vi "Do.vi"(8 "error in":errorcluster, 10 "Actor in":refnum<class "Actor.lvclass">, 11 "Stop Calibration":refnum<class "Send Stop Calibration MSG.lvclass">) -> (0 "error out":errorcluster, 2 "Actor out":refnum<class "Actor.lvclass">)   [LabVIEW 2014, in "Controller.lvlib" / "Send Stop Calibration MSG.lvclass"]
doc: "(<B>Filename</B>: Actor Framework.lvlib:Message.lvclass:Do.vi)\n\nDefines what a message does when it is received by an actor. Generally, a message instructs an actor to invoke one of its methods. By default, this method does nothing. A child class must override it to define behavior. Create a child class by using the Actor Framework Message Maker dialog box."
uses:
  Send Stop Calibration MSG.lvclass
  <vilib>/ActorFramework/Actor/Actor.lvclass
  Controller.lvclass
  Calibration/Send External Stop MSG/Send External Stop MSG.lvclass
  Controls/eMap.ctl
  <vilib>/ActorFramework/Message Enqueuer/Message Enqueuer.lvclass
  SuperActor/SuperActor.lvclass/SuperActor.ctl
  <vilib>/ActorFramework/Message Enqueuer/Message Enqueuer.lvclass/Message Enqueuer.ctl
  SuperActor/Read Log Session.vi
  <vilib>/ActorFramework/Message Priority Queue/Priority Enqueue.vi
  <userlib>/_Session Fwk/Session - Root.lvclass
  reusable/Session APIs/Session Log/System Log.lvclass
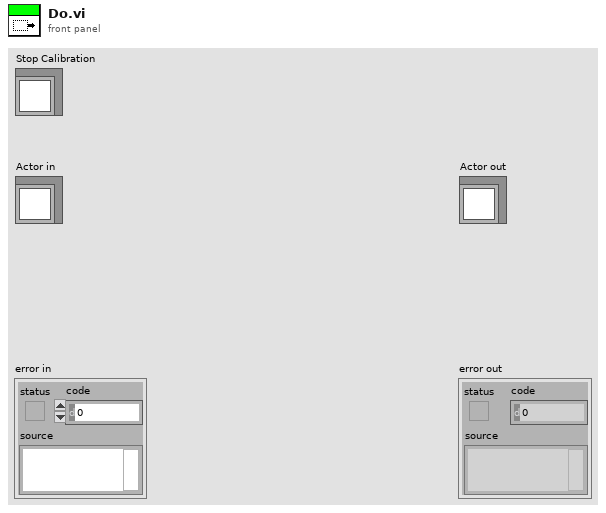
[diagram p1: front panel]
types:
  T1 = typedef "Controller.lvlib/Controller.lvclass/eMap.ctl" = cluster{"Enqueuer":refnum<class "Message Enqueuer.lvclass">, "Active":bool}
  T2 = typedef "Session - Root.lvclass/Session Handle.ctl" = refnum<data-value>
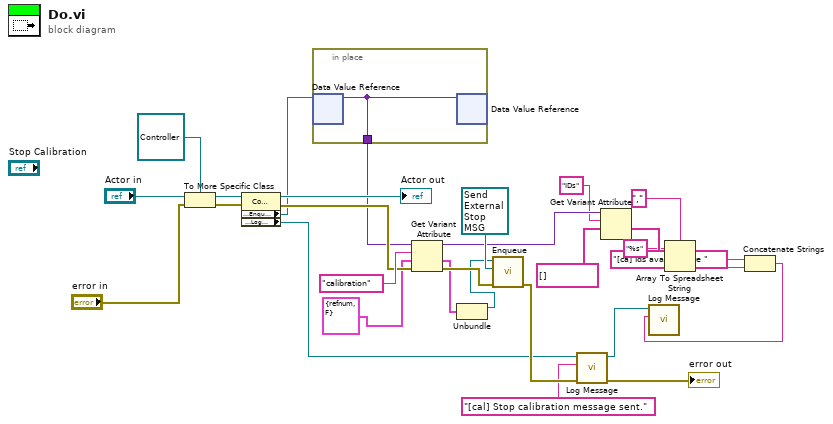
[diagram p0: block diagram]
diagram:
  n1 = To More Specific Class(target class=refnum<class "Controller.lvclass"> refnum ("Controller:Controller"), reference="Actor in", error in="error in") -> (specific class reference=w26:refnum<class "Controller.lvclass">, error out=w24:errorcluster)
  n2 = property class="Controller"(reference=w26, error in=w24) -> (reference out=→"Actor out":refnum<class "Controller.lvclass">, error out=w22:errorcluster, "Accessors:Enqueuer MAP DVR"=w12:refnum<data-value>, "Accessors:Log Session"=w16:T2)
  n3 = in-place {
    in-place-border: [w30] -> w11
    n4 = in-place-dvr #1(w12) -> (w30:variant)  [unwired: 1 out]
    n5 = in-place-dvr #1(w30) -> ()  [unwired: 2 out]
  }
  n6 = Get Variant Attribute(Variant=w11, name="calibration", default value (empty Variant)=T1 {"Enqueuer"=refnum, "Active"=FALSE} ("eMap"), error in=w22) -> (duplicate Variant=w9:variant, value=w14:T1, error out=w20:errorcluster)  [unwired: 1 out]
  n7 = Unbundle(w14) -> ("Enqueuer"=w13:refnum<class "Message Enqueuer.lvclass">)  [unwired: 1 out]
  n8 = call <vilib>:"Enqueue.vi"("error in (no error)"=w20, "Message"=refnum<class "Send External Stop MSG.lvclass"> refnum ("Calibration.lvlib:Send External Stop MSG.lvclass"), "Message Enqueuer in"=w13) -> ("error out"=w19:errorcluster)  [unwired: 7 in, 1 out]
  n9 = call "Log Message.vi"("error in"=w19, "MSG In"="[cal] Stop calibration message sent.", "session in"=w16) -> ("error out"=→"error out":errorcluster, "session out"=w10:T2)  [unwired: 7 in]
  n10 = Get Variant Attribute(Variant=w9, name="IDs", default value (empty Variant)=string[] []) -> (value=w6:string[])  [unwired: 1 in, 3 out]
  n11 = Array To Spreadsheet String(delimiter (Tab)=",", array=w6, 3:"%s" ("format string")) -> (spreadsheet string=w3:string)
  n12 = Concatenate Strings("[ca] Ids available are " ("string"), w3) -> (w1:string)
  n13 = call "Log Message.vi"("MSG In"=w1, "session in"=w10) -> ()  [unwired: 8 in, 2 out]
